vi "ErrorToDb.vi"(0 "reference in":refnum<class "Device.lvclass">, 11 "error in (no error)":errorcluster) -> (4 "reference out":refnum<class "Device.lvclass">, 15 "error out":errorcluster)   [LabVIEW 2019, in "Device.lvclass"]
uses:
  Device.lvclass
  D:/GIT H4000/H4000/src/Proccess_class/Proccess.lvclass
  Proccess_class/Proccess.lvclass/Proccess.ctl
  Logger_class/EventData.ctl
  TypeDef/AlarmType.ctl
  d458cff9-8e45-4544-91af-cfa5b3c8a69c.vi
  Logger_class/Logger.lvclass
  Proccess_class/Proccess.lvclass
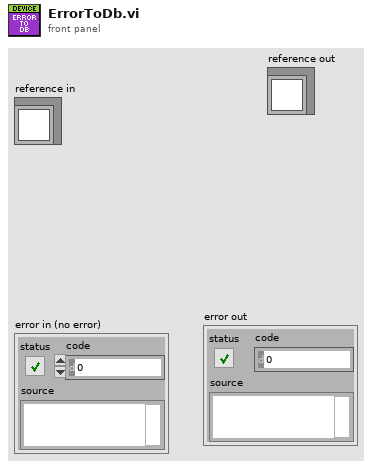
[diagram p1: front panel]
types:
  T1 = typedef "EventData.ctl" = cluster{"obj_tag":string, "event_tag":string, "Description":string, "ALARM TYPE":T2, "Value DBL":dbl, "Value INT":i32, "Value STR":string, "Time Stamp":timestamp}
  T2 = typedef "AlarmType.ctl" = enum16{"Normal", "Warning", "Alarm"}
  T3 = typedef "Proccess.lvclass/TAGs.ctl" = cluster{"TAG":string, "PTAG":string, "DESC":string}
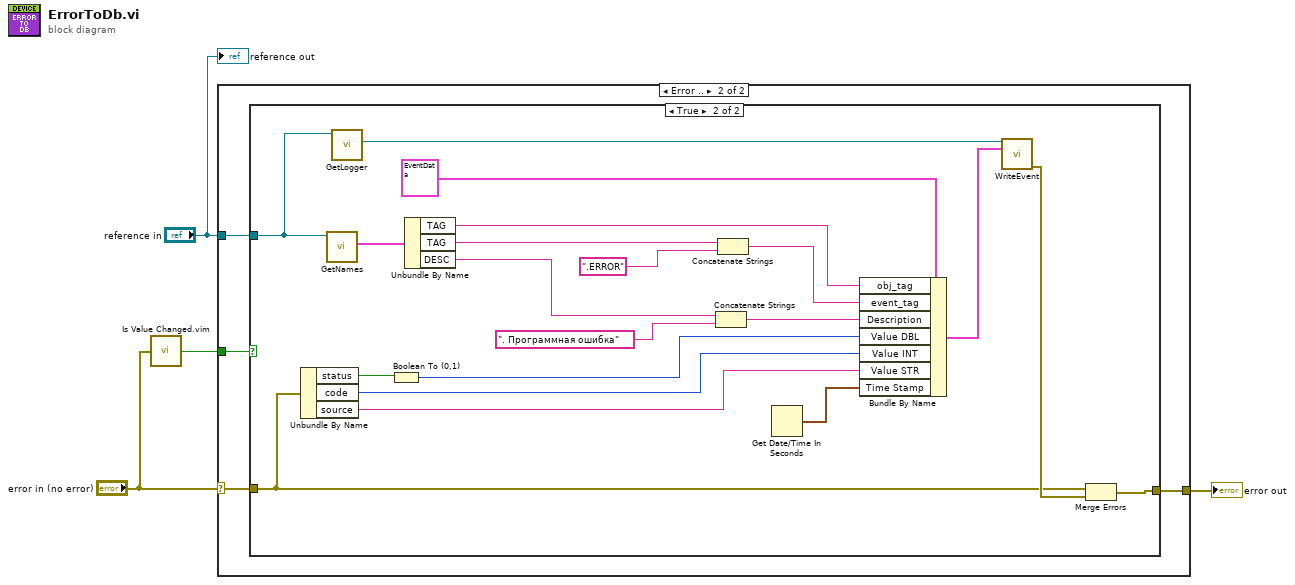
[diagram p0: block diagram]
diagram:
  n1 = call "Is Value Changed.vim"("value"="error in (no error)") -> ("changed or first call?"=w2:bool)
  n2 = case shown="Error .." "error in (no error)" {
    selector: "error in (no error)" -> [w5 w6]
    tunnel: [w5 w9] -> w4
    tunnel: "reference in" -> [_ w8]
    tunnel: w2 -> [_ w7]
    frame No Error {
    }
    frame Error {
      n3 = case shown="True" w7 {
        tunnel: [w10 w12] -> w9
        tunnel: w8 -> [_ w29]
        tunnel: w6 -> [w10 w11]
        frame False {
        }
        frame True {
          n4 = Unbundle By Name(w11) -> ("status"=w16:bool, "code"=w14:i32, "source"=w13:string)
          n5 = call "GetNames.vi"("Proccess in"=w29) -> ("Tags"=w24:T3)  [unwired: 10 in]
          n6 = call "GetLogger.vi"("Proccess in"=w29) -> ("Logger"=w25:refnum<class "Logger.lvclass">)  [unwired: 10 in]
          n7 = Boolean To (0,1)(Boolean=w16) -> (0, 1=w15:i16)
          n8 = Unbundle By Name(w24) -> ("TAG"=w23:string, "TAG"=w22:string, "DESC"=w21:string)
          n9 = Concatenate Strings(w21, ". Программная ошибка" ("string")) -> (w19:string)
          n10 = Concatenate Strings(w22, ".ERROR" ("string")) -> (w27:string)
          n11 = Get Date/Time In Seconds() -> (seconds since 1Jan1904=w20:timestamp)
          n12 = Bundle By Name(cluster=T1 {"obj_tag"="", "event_tag"="", "Description"="", "ALARM TYPE"=enum."Alarm", "Value DBL"=0.0, "Value INT"=0, "Value STR"="", "Time Stamp"=timestamp(0 s since 1904-01-01)} ("Event"), "obj_tag"=w23, "event_tag"=w27, "Description"=w19, "Value DBL"=w15, "Value INT"=w14, "Value STR"=w13, "Time Stamp"=w20) -> (w28:T1)
          n13 = call "WriteEvent.vi"("reference in"=w25, "Event"=w28) -> ("error out"=w30:errorcluster)  [unwired: 12 in, 1 out]
          n14 = Merge Errors(w11, w30) -> (w12:errorcluster)
        }
      }
    }
  }
  "error out" <- w4
  "reference out" <- "reference in"
